vi "Write SPI Configuration.vi"(8 "error in (no error)":errorcluster, 10 "SPI Configuration":T1, 11 "LINX SPI in":refnum<class "LINX SPI.lvclass">) -> (0 "error out":errorcluster, 3 "LINX SPI out":refnum<class "LINX SPI.lvclass">)   [LabVIEW 2020, in "LINX SPI.lvclass"]
uses:
  LINX SPI.lvclass
  <vilib>/MakerHub/LINX/Private/Type Defs/Peripherals/SPI/SPI Bit Order.ctl
  <vilib>/MakerHub/LINX/LMH-LINX.lvlib
  <vilib>/MakerHub/LINX/Private/Type Defs/Peripherals/SPI/SPI Mode.ctl
  <vilib>/MakerHub/LINX/Private/Type Defs/Peripherals/SPI/SPI Configuration.ctl
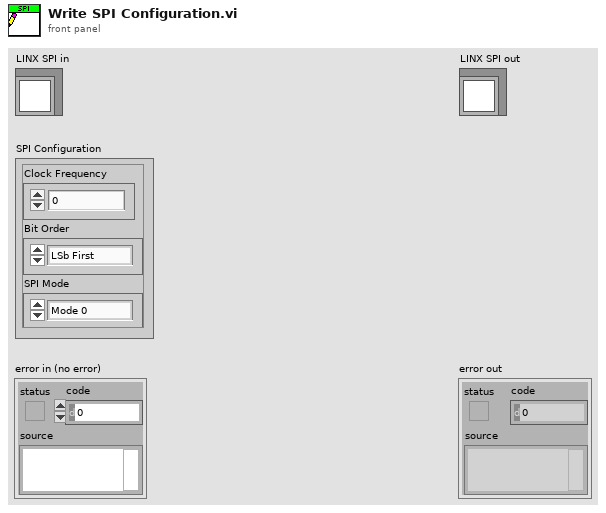
[diagram p1: front panel]
types:
  T1 = typedef "LMH-LINX.lvlib/SPI Configuration.ctl" = cluster{"Clock Frequency":u32, "Bit Order":T2, "SPI Mode":T3}
  T2 = typedef "LMH-LINX.lvlib/SPI Bit Order.ctl" = enum8{"LSb First", "MSb First"}
  T3 = typedef "LMH-LINX.lvlib/SPI Mode.ctl" = enum8{"Mode 0", "Mode 1", "Mode 2", "Mode 3"}
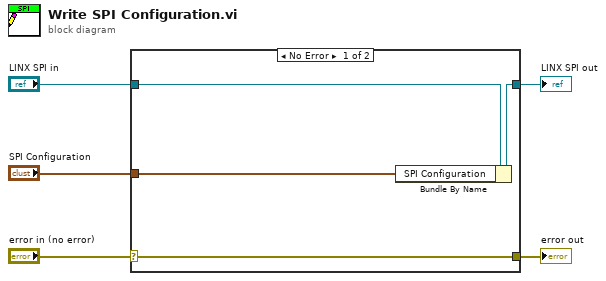
[diagram p0: block diagram]
diagram:
  n1 = case shown="No Error" "error in (no error)" {
    selector: "error in (no error)" -> [w9 w10]
    tunnel: [w9 w10] -> w4
    tunnel: [w7 w11] -> w2
    tunnel: "LINX SPI in" -> [w8 w11]
    tunnel: "SPI Configuration" -> [w6 _]
    frame No Error {
      n2 = Bundle By Name(cluster=w8, "SPI Configuration"=w6) -> (w7:refnum<class "LINX SPI.lvclass">)
    }
    frame Error {
    }
  }
  "error out" <- w4
  "LINX SPI out" <- w2
